vi "3.1_PH.vi"() -> ()   [LabVIEW 2023]
panel:
  out "Liczby losowe":dbl(graph)
  in  "stop":bool
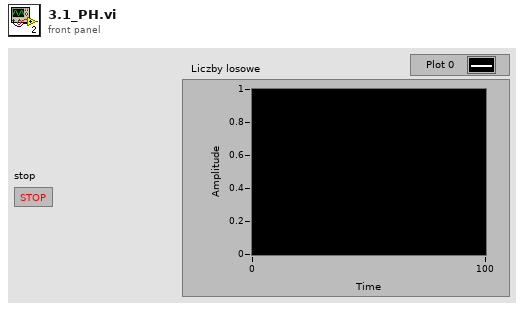
[diagram p1: front panel]
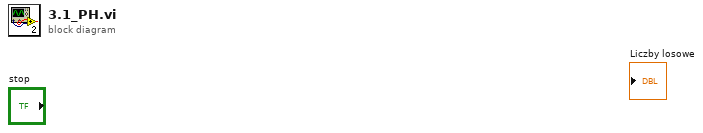
[diagram p0: block diagram]
diagram:
